vi "formatFileData.vi"(8 "error in (no error)":errorcluster, 11 "message out":T1) -> (0 "error out":errorcluster, 3 "LogData":string)   [LabVIEW 2017, in "loggingModule.lvlib"]
doc: "This VI formats the data and creates a string to save in the log.\n\nThe string is formatted as follows:\n\ntimestamp; calling module; message; error number; error source"
uses:
  loggingModule.lvlib
  Queue/TypeDefs/message.ctl
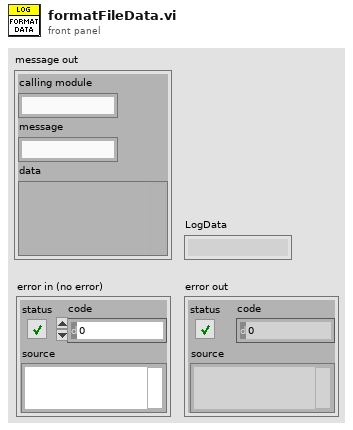
[diagram p1: front panel]
types:
  T1 = typedef "loggingModule.lvlib/message.ctl" = cluster{"calling module":string, "message":string, "data":variant}
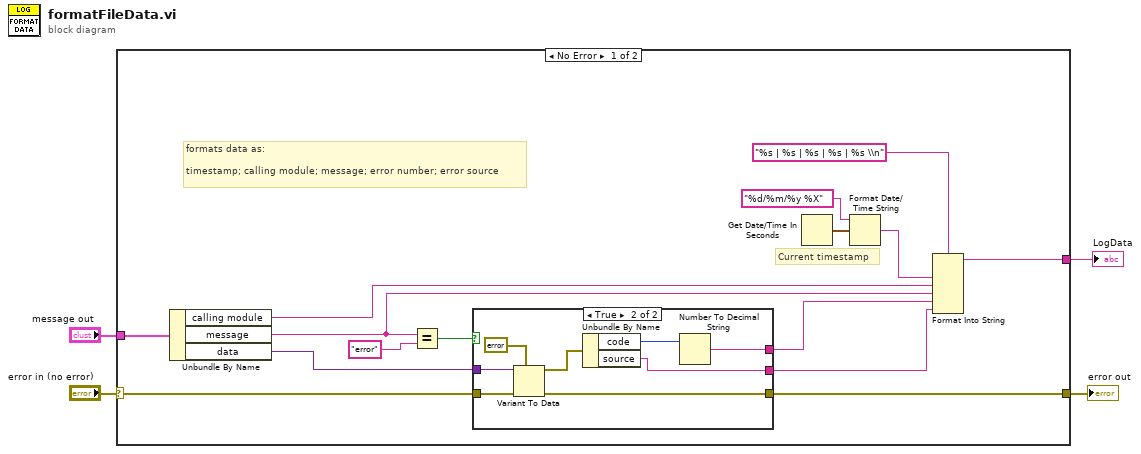
[diagram p0: block diagram]
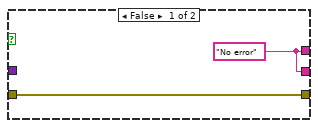
[diagram p2: hidden frame]
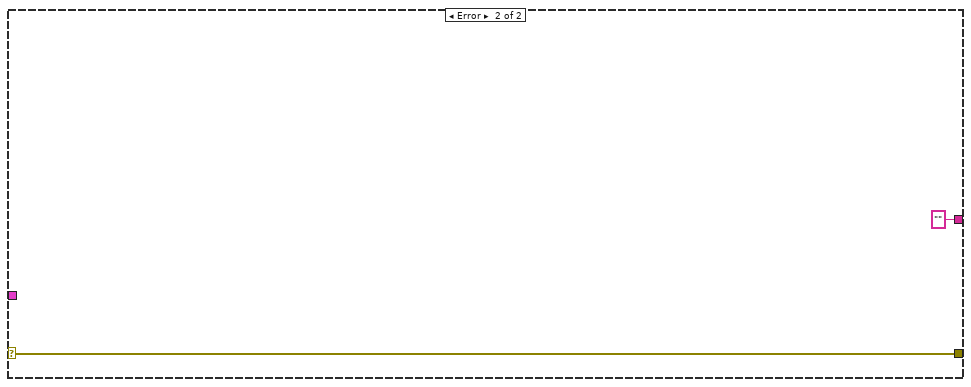
[diagram p3: hidden frame]
diagram:
  n1 = case shown="No Error" "error in (no error)" {
    selector: "error in (no error)" -> [w10 w31]
    tunnel: [w9 w31] -> w3
    tunnel: "message out" -> [w19 _]
    tunnel: [w12 ""] -> w1
    frame No Error {
      # "formats data as:\n\ntimestamp; calling module; message; error number; error source"
      # "Current timestamp"
      n2 = Unbundle By Name(w19) -> ("calling module"=w15:string, "message"=w14:string, "data"=w11:variant)
      n3 = Equal?(x=w14, y="error") -> (x = y?=w8:bool)
      n4 = case shown="True" w8 {
        tunnel: w11 -> [_ w29]
        tunnel: w10 -> [w21 w27]
        tunnel: [w21 w26] -> w9
        tunnel: [w20 w23] -> w7
        tunnel: [w20 w22] -> w6
        frame False {
          w20 = "No error"
        }
        frame True {
          n5 = Variant To Data(error in=w27, type=errorcluster {"status"=FALSE, "code"=0, "source"=""} ("error constant"), Variant=w29) -> (data=w25:errorcluster, error out=w26:errorcluster)
          n6 = Unbundle By Name(w25) -> ("code"=w24:i32, "source"=w22:string)
          n7 = Number To Decimal String(number=w24) -> (decimal integer string=w23:string)  [unwired: 1 in]
        }
      }
      n8 = Get Date/Time In Seconds() -> (seconds since 1Jan1904=w18:timestamp)
      n9 = Format Date/Time String(time format string (%c)="%d/%m/%y %X", seconds (now)=w18) -> (date/time string=w16:string)  [unwired: 1 in]
      n10 = Format Into String(format string="%s | %s | %s | %s | %s \\n", w16, w15, w14, w7, w6) -> (resulting string=w12:string)  [unwired: 2 in, 1 out]
    }
    frame Error {
    }
  }
  "error out" <- w3
  "LogData" <- w1
